vi "Configure Modulation Waveform.vi"   [LabVIEW 2012, in "Agilent PSG MXG Series.lvlib"]
doc: "Configures parameters for noise, ramp, dual-sine or swept-sine waveform."
uses:
  <instrlib>/Agilent PSG MXG Series/Agilent PSG MXG Series.lvlib
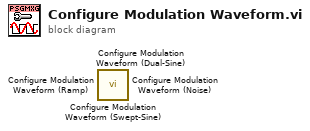
[diagram p0: block diagram]
diagram:
  n1 = call <instrlib>:"Configure Modulation Waveform (Swept-Sine).vi"() -> ()  [unwired: 10 in, 2 out]
  n2 = call <instrlib>:"Configure Modulation Waveform (Dual-Sine).vi"() -> ()  [unwired: 10 in, 2 out]
  n3 = call <instrlib>:"Configure Modulation Waveform (Ramp).vi"() -> ()  [unwired: 10 in, 2 out]
  n4 = call <instrlib>:"Configure Modulation Waveform (Noise).vi"() -> ()  [unwired: 10 in, 2 out]
